vi "Main.vi"(11 "Module Admin":refnum<class "Delacor_lib_QMH_Module Admin.lvclass">) -> ()   [LabVIEW 2021, in "Control Panel.lvlib"]
doc: "This template is based off of the Queued Message Handler design pattern and the Queued Message Handler project template that ships with LabVIEW.\n\nThe main difference is that the queue is private to this module and communication between modules is performed via Broadcast and Request events.\n\nRequest events are wrapped in public API methods and are handled in the Event Handling Loop (EHL) of this VI. Any module can register for Broadcast events sent by this module. The EHL generates messages based on user interface actions.\n\nThe Message Handling Loop (MHL) processes messages generated by the EHL, or by other messages. The messages are string values, so new messages can be added easily to the Message Cases case structure in the MHL. Each message cluster can also provide an optional value for Message Data, which is a variant that can be converted to whatever message-specific data is required.\n_____\nBased on DQMH Project Template 7.0.1.1316."
uses:
  Control Panel.lvlib
  <vilib>/Delacor/Delacor QMH/Libraries/Message Queue_class/Delacor_lib_QMH_Message Queue.lvclass
  Module Data--cluster.ctl
  <vilib>/Delacor/Delacor QMH/Libraries/Message Queue_class/Delacor_lib_QMH_Enqueue Message (Single).vi
  Stop Argument--cluster.ctl
  <vilib>/Delacor/Delacor QMH/Libraries/Module Admin_class/Delacor_lib_QMH_Module Admin.lvclass
  PS/PS.lvlib
  DAQ/DAQ.lvlib
  SCOPE/SCOPE.lvlib
  Panel Load Argument--cluster.ctl
panel:
  in  "Options":i32(listbox)
  out "error out":errorcluster
  out "Status":string
  in  "Simulate MHL Error":bool
  in  "Simulate EHL Error":bool
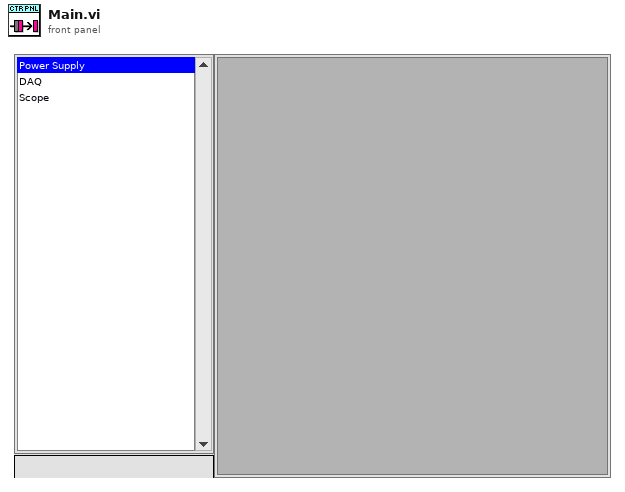
[diagram p1: front panel]
types:
  T1 = typedef "Control Panel.lvlib/Broadcast Events--cluster.ctl" = cluster{"Module Did Init":refnum<user-event>, "Status Updated":refnum<user-event>, "Error Reported":refnum<user-event>, "Module Did Stop":refnum<user-event>, "Update Module Execution Status":refnum<user-event>}
  T2 = typedef "PS.lvlib/Broadcast Events--cluster.ctl" = cluster{"Module Did Init":refnum<user-event>, "Status Updated":refnum<user-event>, "Error Reported":refnum<user-event>, "Module Did Stop":refnum<user-event>, "Update Module Execution Status":refnum<user-event>}
  T3 = typedef "DAQ.lvlib/Broadcast Events--cluster.ctl" = cluster{"Module Did Init":refnum<user-event>, "Status Updated":refnum<user-event>, "Error Reported":refnum<user-event>, "Module Did Stop":refnum<user-event>, "Update Module Execution Status":refnum<user-event>}
  T4 = typedef "SCOPE.lvlib/Broadcast Events--cluster.ctl" = cluster{"Module Did Init":refnum<user-event>, "Status Updated":refnum<user-event>, "Error Reported":refnum<user-event>, "Module Did Stop":refnum<user-event>, "Update Module Execution Status":refnum<user-event>}
  T5 = typedef "Control Panel.lvlib/Request Events--cluster.ctl" = cluster{"Stop Module":refnum<user-event>, "Show Panel":refnum<user-event>, "Hide Panel":refnum<user-event>, "Get Module Execution Status":refnum<user-event>, "Show Diagram":refnum<user-event>, "Private":cluster{"Panel Load":refnum<user-event>}}
  T6 = typedef "Control Panel.lvlib/Module Data--cluster.ctl" = cluster{"Status":string}
  T7 = enum32{"invalid lock state", "Not Locked", "Locked (No Password)", "Password-protected"}
  T8 = typedef "Control Panel.lvlib/Stop Argument--cluster.ctl" = cluster{"Origin":string, "Exit via Stop Module Req?":bool, "Wait for Module to stop?":bool}
  T9 = typedef "Control Panel.lvlib/Panel Load Argument--cluster.ctl" = cluster{"Panel Index":i32}
  T10 = enum32{"Invalid", "Standard", "Closed", "Hidden", "Minimized", "Maximized"}
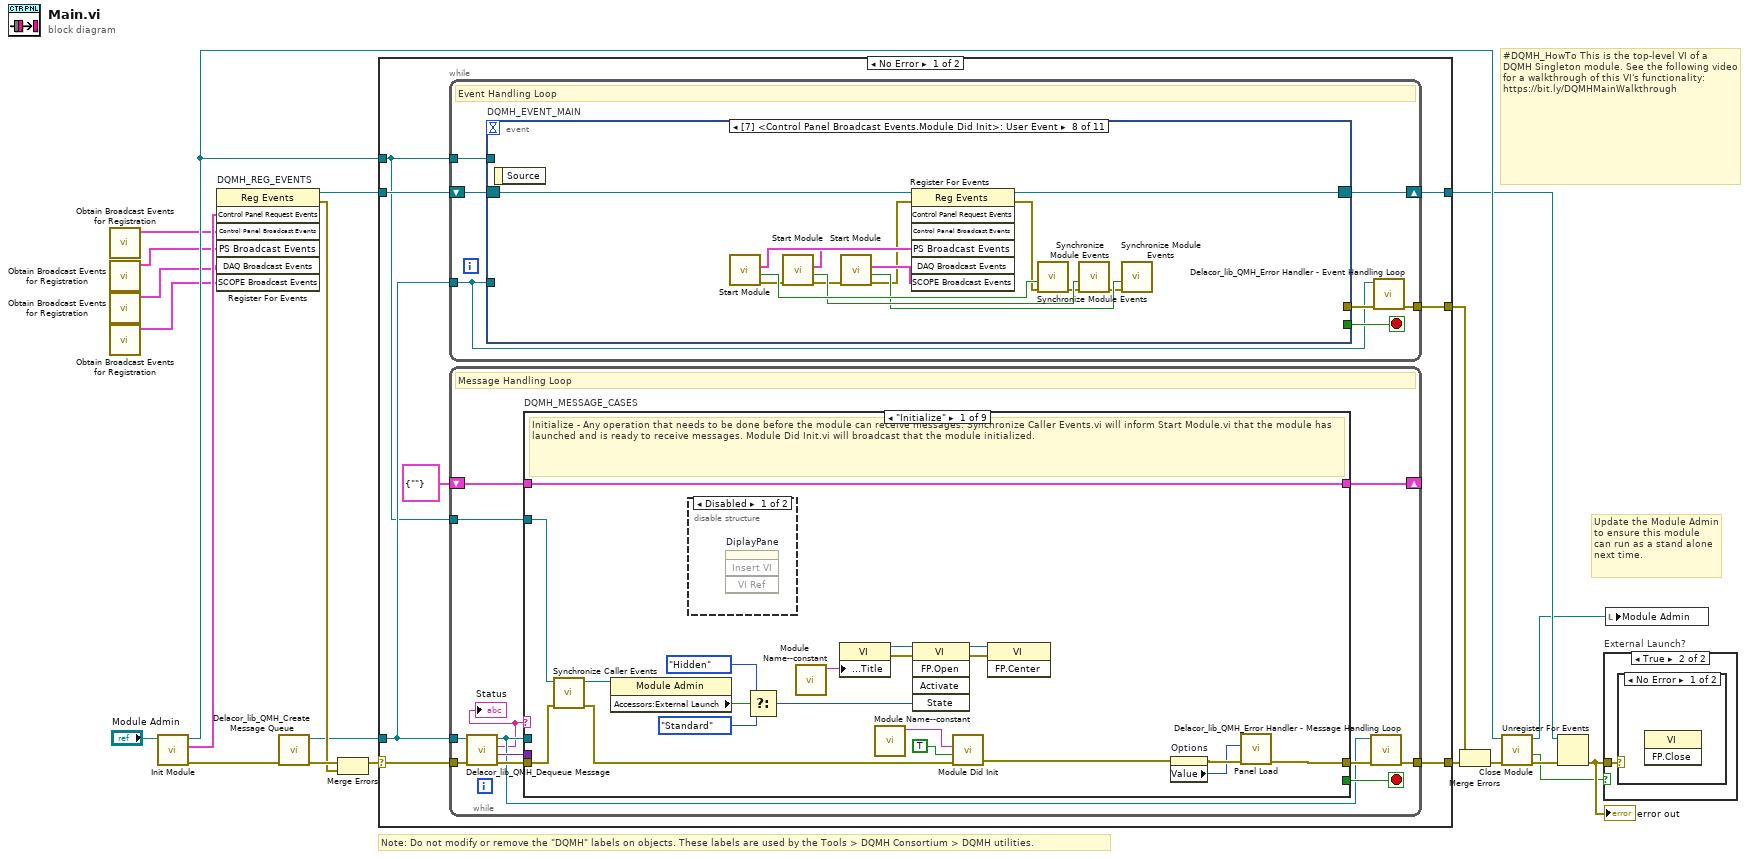
[diagram p0: block diagram]
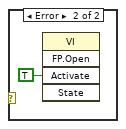
[diagram p3: hidden frame]
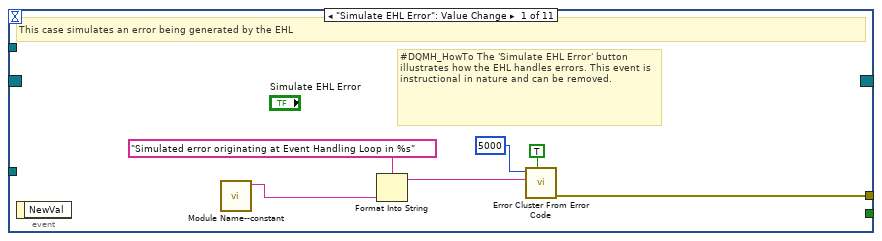
[diagram p4: hidden frame]
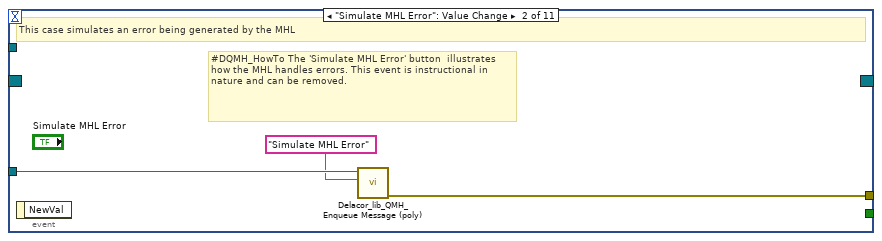
[diagram p5: hidden frame]
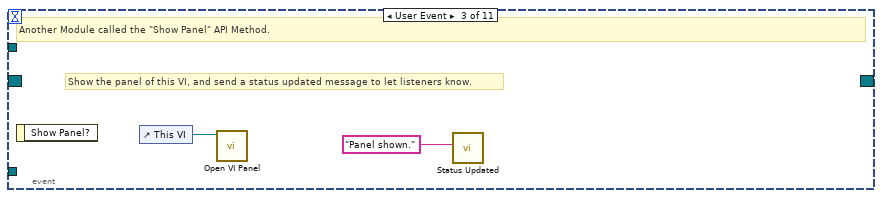
[diagram p6: hidden frame]
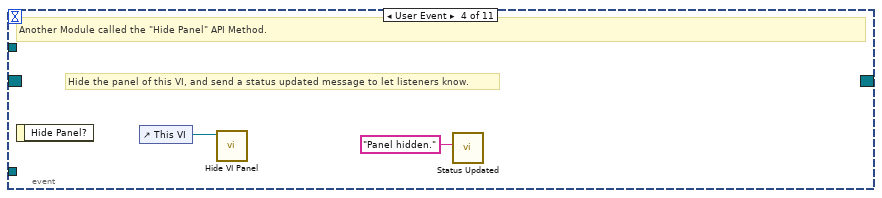
[diagram p7: hidden frame]
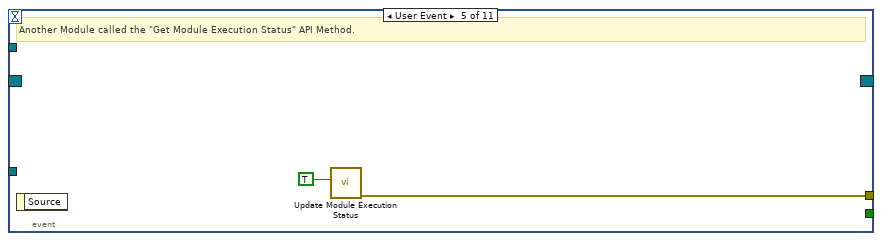
[diagram p8: hidden frame]
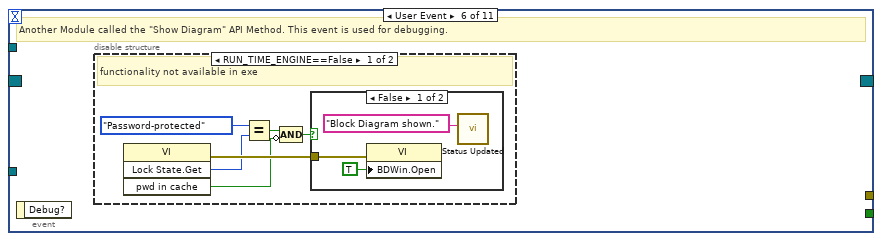
[diagram p9: hidden frame]
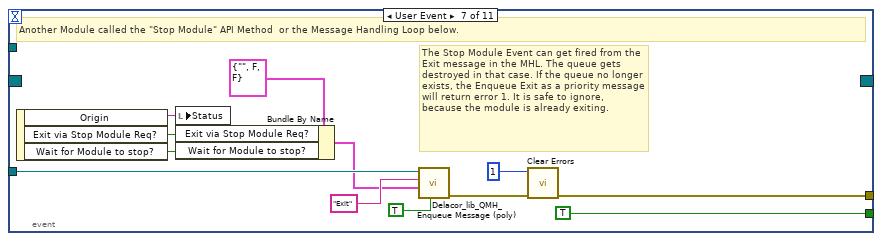
[diagram p12: hidden frame]
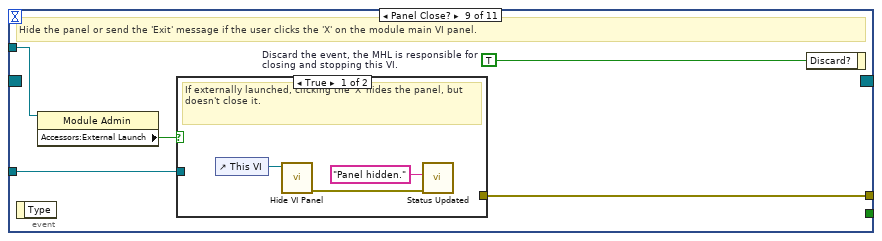
[diagram p13: hidden frame]
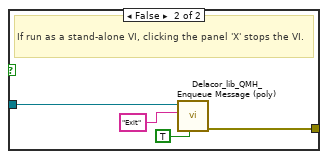
[diagram p14: hidden frame]
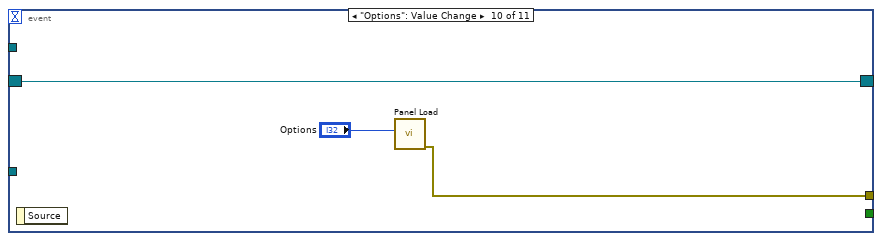
[diagram p15: hidden frame]
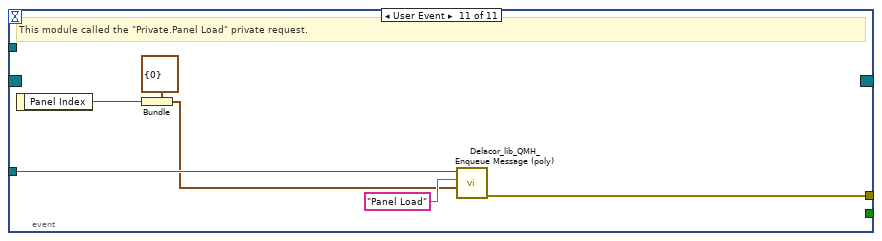
[diagram p16: hidden frame]
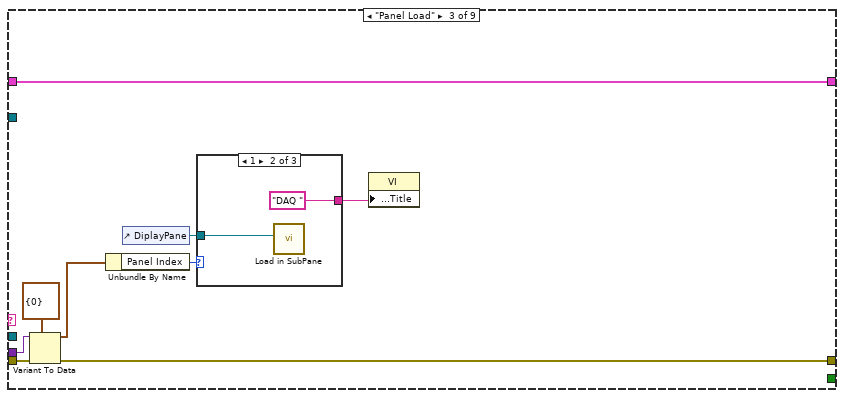
[diagram p19: hidden frame]
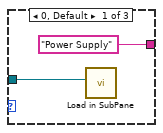
[diagram p20: hidden frame]
diagram:
  # "#DQMH_HowTo This is the top-level VI of a DQMH Singleton module. See the following video for a walkthrough of this VI's functionality: https://bit.ly/DQMHMainWalkthrough"
  # "Note: Do not modify or remove the \"DQMH\" labels on objects. These labels are used by the Tools > DQMH Consortium > DQMH utilities."
  # "Update the Module Admin to ensure this module can run as a stand alone next time."
  n1 = call "Obtain Broadcast Events for Registration.vi"() -> ("Control Panel Broadcast Events"=w4:T1)  [unwired: 9 in, 2 out]
  n2 = call "Obtain Broadcast Events for Registration.vi"() -> ("PS Broadcast Events"=w3:T2)  [unwired: 9 in, 2 out]
  n3 = call "Obtain Broadcast Events for Registration.vi"() -> ("DAQ Broadcast Events"=w2:T3)  [unwired: 9 in, 2 out]
  n4 = call "Obtain Broadcast Events for Registration.vi"() -> ("SCOPE Broadcast Events"=w1:T4)  [unwired: 9 in, 2 out]
  n5 = call "Init Module.vi"("Singleton Module Admin in"="Module Admin") -> ("error out"=w20:errorcluster, "Control Panel Request Events"=w9:T5, "Singleton Module Admin out"=w12:refnum<class "Delacor_lib_QMH_Module Admin.lvclass">)  [unwired: 8 in]
  n6 = register-events "DQMH_REG_EVENTS"(w9, w4, w3, w2, w1) -> (reference out=w10:refnum<event-registration>, error out=w13:errorcluster)  [unwired: 2 in]
  n7 = call <vilib>:"Delacor_lib_QMH_Create Message Queue.vi"("error in"=w20) -> ("error out"=w15:errorcluster, "Message Queue"=w8:refnum<class "Delacor_lib_QMH_Message Queue.lvclass">)  [unwired: 9 in]
  n8 = Merge Errors(w15, w13) -> (w14:errorcluster)
  n9 = case shown="No Error" w14 {
    selector: w14 -> [w27 w224]
    tunnel: [w29 w223] -> w21
    tunnel: [w26 w222] -> w11
    tunnel: w10 -> [w24 w222]
    tunnel: w8 -> [w23 w217]
    tunnel: [w28 _] -> w18
    tunnel: w12 -> [w22 w218]
    frame No Error {
      n10 = while {
        tunnel: w23 -> [w30]
        shift-right: [w33] -> w26
        shift-left: w24 -> [w34]
        tunnel: [w35] -> w28
        tunnel: w22 -> [w31]
        stop <- w32 stop-if-true
        # "Event Handling Loop"
        n11 = event "DQMH_EVENT_MAIN" shown="[7] <Control Panel Broadcast Events.Module Did Init>: User Event" {
          selector: w34 -> [_ _ _ _ _ _ _ w74 _ w101 _]
          dyn-events: [_ _ _ _ _ _ _ w73 _ w101 _] -> w33
          timeout: _ -> [_ _ _ _ _ _ _ _ _ _ _]
          tunnel: [_ _ _ _ _ _ TRUE ("Discard?") _ _ _ _] -> w32
          tunnel: w30 -> [_ w44 _ _ _ _ w68 _ w89 _ w107]
          tunnel: [w42 w45 _ _ w51 _ w71 _ w91 w99 w102] -> w36
          tunnel: w31 -> [_ _ _ _ _ _ _ _ w88 _ _]
          event "Simulate EHL Error": Value Change {
            # "#DQMH_HowTo The 'Simulate EHL Error' button  illustrates how the EHL handles errors. This event is instructional in nature and can be removed."
            # "This case simulates an error being generated by the EHL"
            n12 = event-data() -> ()  [unwired: 1 in, 1 out]
            n13 = call "Module Name--constant.vi"() -> ("Module Name"=w39:string)  [unwired: 11 in]
            n14 = Format Into String(format string="Simulated error originating at Event Handling Loop in %s", w39) -> (resulting string=w40:string)  [unwired: 2 in, 1 out]
            n15 = call <vilib>:"Error Cluster From Error Code.vi"("show call chain? (False)"=TRUE, "error message (\"\")"=w40, "error code (0)"=5000) -> ("error out"=w42:errorcluster)  [unwired: 6 in]
          }
          event "Simulate MHL Error": Value Change {
            # "#DQMH_HowTo The 'Simulate MHL Error' button  illustrates how the MHL handles errors. This event is instructional in nature and can be removed."
            # "This case simulates an error being generated by the MHL"
            n16 = event-data() -> ()  [unwired: 1 in, 1 out]
            n17 = call-poly <vilib>:"Delacor_lib_QMH_Enqueue Message (poly).vi"("Message"="Simulate MHL Error", "Message Queue in"=w44) -> ("error out"=w45:errorcluster)  [unwired: 8 in, 1 out]
          }
          event User Event {
            # "Show the panel of this VI, and send a status updated message to let listeners know."
            # "Another Module called the \"Show Panel\" API Method."
            n18 = event-data() -> ()  [unwired: 1 in, 1 out]
            n19 = control-ref of="This VI"() -> (w47:refnum<vi>)
            n20 = call "Open VI Panel.vi"("VI"=w47) -> ()  [unwired: 10 in, 1 out]
            n21 = call "Status Updated.vi"("Status"="Panel shown." ("format string")) -> ()  [unwired: 10 in, 1 out]
          }
          event User Event {
            # "Hide the panel of this VI, and send a status updated message to let listeners know."
            # "Another Module called the \"Hide Panel\" API Method."
            n22 = event-data() -> ()  [unwired: 1 in, 1 out]
            n23 = control-ref of="This VI"() -> (w49:refnum<vi>)
            n24 = call "Hide VI Panel.vi"("VI"=w49) -> ()  [unwired: 10 in, 1 out]
            n25 = call "Status Updated.vi"("Status"="Panel hidden." ("format string")) -> ()  [unwired: 10 in, 1 out]
          }
          event User Event {
            # "Another Module called the \"Get Module Execution Status\" API Method."
            n26 = event-data() -> ()  [unwired: 1 in, 1 out]
            n27 = call "Update Module Execution Status.vi"("Running?"=TRUE) -> ("error out"=w51:errorcluster)  [unwired: 10 in]
          }
          event User Event {
            # "Another Module called the \"Show Diagram\" API Method. This event is used for debugging."
            n28 = event-data() -> ()  [unwired: 1 in, 1 out]
            n29 = disable-structure shown="RUN_TIME_ENGINE==False" {
              frame condition #0 (active) {
                # "functionality not available in exe"
                n30 = invoke on="Invoke Node" class="VI" method="Lock State.Get"() -> (error out=w57:errorcluster, "Get Lock State"=w56:T7, "pwd in cache"=w53:bool)  [unwired: 4 in, 1 out]
                n31 = Equal?(x=T7."Password-protected", y=w56) -> (x = y?=w54:bool)
                n32 = Compound Arithmetic op=AND(w54, invert w53) -> (w52:bool)
                n33 = case shown="False" w52 {
                  tunnel: w57 -> [w60 _]
                  frame False {
                    n34 = property on="Property Node" class="VI"(error in=w60, "BDWin.Open"=TRUE ("Block Diagram Window:Open")) -> ()  [unwired: 1 in, 2 out]
                    n35 = call "Status Updated.vi"("Status"="Block Diagram shown." ("format string")) -> ()  [unwired: 10 in, 1 out]
                  }
                  frame True {
                    # "Password-protected VI, and the password is not in the cache. Do not show the diagram."
                  }
                }
              }
              frame condition #1 {
              }
            }
          }
          event User Event {
            # "The Stop Module Event can get fired from the Exit message in the MHL. The queue gets destroyed in that case. If the queue no longer exists, the Enqueue Exit as a priority message will return error 1. It is safe to ignore, because the module is already exiting."
            # "Another Module called the \"Stop Module\" API Method  or the Message Handling Loop below."
            n36 = event-data() -> ("Origin"=w67:string, "Exit via Stop Module Req?"=w63:bool, "Wait for Module to stop?"=w62:bool)  [unwired: 1 in]
            n37 = local write "Status"(w67) -> ()
            n38 = Bundle By Name(cluster=T8 {"Origin"="", "Exit via Stop Module Req?"=FALSE, "Wait for Module to stop?"=FALSE} ("Stop Argument"), "Exit via Stop Module Req?"=w63, "Wait for Module to stop?"=w62) -> (w61:T8)
            n39 = call-poly <vilib>:"Delacor_lib_QMH_Enqueue Message (poly).vi"("Priority Message? (F)"=TRUE, "Message Data"=w61, "Message"="Exit", "Message Queue in"=w68) -> ("error out"=w72:errorcluster)  [unwired: 6 in, 1 out]
            n40 = call <vilib>:"Clear Errors.vi"("error in (no error)"=w72, "specific error code to clear (0: all)"=1) -> ("error out"=w71:errorcluster)  [unwired: 4 in, 1 out]
          }
          event User Event {
            n41 = event-data() -> ()  [unwired: 1 in, 1 out]
            n42 = call "Start Module.vi"() -> ("error out"=w80:errorcluster, "Wait for Event Sync?"=w86:bool, "PS Broadcast Events"=w83:T2)  [unwired: 8 in, 1 out]
            n43 = call "Start Module.vi"("error in (no error)"=w80) -> ("error out"=w79:errorcluster, "Wait for Event Sync?"=w85:bool, "SCOPE Broadcast Events"=w82:T4)  [unwired: 7 in, 1 out]
            n44 = call "Start Module.vi"("error in (no error)"=w79) -> ("error out"=w78:errorcluster, "Wait for Event Sync?"=w84:bool, "DAQ Broadcast Events"=w81:T3)  [unwired: 7 in, 1 out]
            n45 = register-events(reference=w74, error in=w78, w83, w82, w81) -> (reference out=w73:refnum<event-registration>, error out=w77:errorcluster)  [unwired: 2 in]
            n46 = call "Synchronize Module Events.vi"("error in (no error)"=w77, "Wait for Event Sync?"=w86) -> ("error out"=w75:errorcluster)  [unwired: 9 in]
            n47 = call "Synchronize Module Events.vi"("error in (no error)"=w75, "Wait for Event Sync?"=w85) -> ("error out"=w76:errorcluster)  [unwired: 9 in]
            n48 = call "Synchronize Module Events.vi"("error in (no error)"=w76, "Wait for Event Sync?"=w84) -> ()  [unwired: 9 in, 1 out]
          }
          event Panel Close? {
            w90 = TRUE  # Discard the event, the MHL is responsible for closing and stopping this VI.
            # "Hide the panel or send the 'Exit' message if the user clicks the 'X' on the module main VI panel."
            n49 = event-data() -> ()  [unwired: 1 in, 1 out]
            n50 = property on="Property Node" class="Module Admin"(reference=w88) -> ("Accessors:External Launch"=w87:bool)  [unwired: 1 in, 2 out]
            n51 = case shown="True" w87 {
              tunnel: w89 -> [_ w97]
              tunnel: [_ w98] -> w91
              frame True {
                # "If externally launched, clicking the 'X' hides the panel, but doesn't close it."
                n52 = control-ref of="This VI"() -> (w94:refnum<vi>)
                n53 = call "Hide VI Panel.vi"("VI"=w94) -> ("error out"=w92:errorcluster)  [unwired: 10 in]
                n54 = call "Status Updated.vi"("error in"=w92, "Status"="Panel hidden." ("format string")) -> ()  [unwired: 9 in, 1 out]
              }
              frame False {
                # "If run as a stand-alone VI, clicking the panel 'X' stops the VI."
                n55 = call-poly <vilib>:"Delacor_lib_QMH_Enqueue Message (poly).vi"("Priority Message? (F)"=TRUE, "Message"="Exit", "Message Queue in"=w97) -> ("error out"=w98:errorcluster)  [unwired: 7 in, 1 out]
              }
            }
            n56 = event-data ("Event Filter Node")("Discard?"=w90) -> ()  [unwired: 1 in, 1 out]
          }
          event "Options": Value Change {
            n57 = event-data() -> ()  [unwired: 1 in, 1 out]
            n58 = call "Panel Load.vi"("Panel Index"="Options") -> ("error out"=w99:errorcluster)  [unwired: 10 in]
          }
          event User Event {
            # "This module called the \"Private.Panel Load\" private request."
            n59 = event-data() -> ("Panel Index"=w103:i32)  [unwired: 1 in]
            n60 = Bundle(cluster=T9 {"Panel Index"=0} ("Panel Load Argument"), "Panel Index"=w103) -> (w104:T9)
            n61 = call-poly <vilib>:"Delacor_lib_QMH_Enqueue Message (poly).vi"("Message Data"=w104, "Message"="Panel Load", "Message Queue in"=w107) -> ("error out"=w102:errorcluster)  [unwired: 7 in, 1 out]
          }
        }
        n62 = call-dynamic "Delacor_lib_QMH_Error Handler - Event Handling Loop.vi"("error in"=w36, "Message Queue in"=w30) -> ("dup error in"=w35:errorcluster)  [unwired: 8 in, 1 out]
      }
      n63 = while {
        tunnel: w23 -> [w109]
        shift-right: [w116] -> _
        shift-left: T6 {"Status"=""} ("Data Cluster") -> [w117]
        tunnel: w27 -> [w119]
        tunnel: [w112] -> w29
        tunnel: w22 -> [w113]
        stop <- w115 stop-if-true
        # "Message Handling Loop"
        n64 = call-dynamic "Delacor_lib_QMH_Dequeue Message.vi"("error in"=w119, "Message Queue in"=w109) -> ("error out"=w118:errorcluster, "Message Data"=w114:variant, "Message"=w108:string, "Message Queue out"=w110:refnum<class "Delacor_lib_QMH_Message Queue.lvclass">)  [unwired: 6 in]
        "Status" <- w108
        n65 = case "DQMH_MESSAGE_CASES" shown="\"Initialize\"" w108 {
          selector: w108 -> [_ _ _ _ _ _ _ _ w212]
          tunnel: w110 -> [_ _ _ _ _ _ w174 w200 _]
          tunnel: w118 -> [w137 w141 w150 w159 w161 w170 w181 w206 w215]
          tunnel: [w123 w141 w148 w158 w161 w169 w177 w201 w216] -> w111
          tunnel: w117 -> [w124 w140 w149 w157 w160 w167 w176 w199 w213]
          tunnel: [w124 w140 w149 w157 w160 w167 w176 w199 w213] -> w116
          tunnel: [_ _ _ _ _ _ _ w198 _] -> w115
          tunnel: w114 -> [_ _ w147 _ _ _ w175 w197 _]
          tunnel: w113 -> [w128 _ _ _ _ _ w173 w192 _]
          frame "Initialize" {
            # "Initialize - Any operation that needs to be done before the module can receive messages. Synchronize Caller Events.vi will inform Start Module.vi that the module has launched and is ready to receive messages. Module Did Init.vi will broadcast that the module initialized."
            n66 = call "Synchronize Caller Events.vi"("error in"=w137, "Singleton Module Admin in"=w128) -> ("error out"=w136:errorcluster, "Singleton Module Admin out"=w125:refnum<class "Delacor_lib_QMH_Module Admin.lvclass">)  [unwired: 8 in]
            n67 = property on="Property Node" class="Module Admin"(reference=w125) -> ("Accessors:External Launch"=w132:bool)  [unwired: 1 in, 2 out]
            n68 = disable-structure shown="Disabled" {
              frame Disabled {
                n69 = invoke on="DiplayPane" class="SubPnl" method="Insert VI"() -> ()  [unwired: 4 in, 4 out]
              }
              frame Enabled {
              }
            }
            n70 = Select(t=T10."Hidden" ("State"), s=w132, f=T10."Standard" ("State")) -> (s? t:f=w129:T10)
            n71 = call "Module Name--constant.vi"() -> ("Module Name"=w135:string)  [unwired: 11 in]
            n72 = property on="Property Node" class="VI"("Front Panel.Title"=w135) -> (reference out=w134:refnum<vi>, error out=w139:errorcluster)  [unwired: 2 in]
            n73 = call "Module Name--constant.vi"() -> ("Module Name"=w126:string)  [unwired: 11 in]
            n74 = invoke on="Invoke Node" class="VI" method="FP.Open"(reference=w134, error in=w139, "State"=w129) -> (reference out=w133:refnum<vi>, error out=w138:errorcluster)  [unwired: 2 in, 3 out]
            n75 = call "Module Did Init.vi"("error in"=w136, "Initialized?"=TRUE, "Origin"=w126) -> ("error out"=w122:errorcluster)  [unwired: 8 in]
            n76 = invoke on="Invoke Node" class="VI" method="FP.Center"(reference=w133, error in=w138) -> ()  [unwired: 1 in, 3 out]
            n77 = property on="Options" class="LstBox (strict)"(error in=w122) -> (error out=w121:errorcluster, "Value"=w120:i32)  [unwired: 1 in, 1 out]
            n78 = call "Panel Load.vi"("error in"=w121, "Panel Index"=w120) -> ("error out"=w123:errorcluster)  [unwired: 9 in]
          }
          frame "---Module Specific---" {
            # "Separator -- The following cases handle messages specific to this Module."
          }
          frame "Panel Load" {
            n79 = Variant To Data(error in=w150, type=T9 {"Panel Index"=0} ("Panel Load Argument"), Variant=w147) -> (data=w145:T9, error out=w148:errorcluster)
            n80 = Unbundle By Name(w145) -> ("Panel Index"=w144:i32)
            n81 = control-ref of="DiplayPane"() -> (w143:refnum<vi>)
            n82 = case shown="1" w144 {
              tunnel: w143 -> [w152 w154 w156]
              tunnel: ["Power Supply" "DAQ " "SCOPE"] -> w142
              frame 0, Default {
                n83 = call "Load in SubPane.vi"("Subpanel Ref"=w152) -> ()  [unwired: 10 in, 1 out]
              }
              frame 1 {
                n84 = call "Load in SubPane.vi"("Subpanel Ref"=w154) -> ()  [unwired: 10 in, 1 out]
              }
              frame 2 {
                n85 = call "Load in SubPane.vi"("Subpanel Ref"=w156) -> ()  [unwired: 10 in, 1 out]
              }
            }
            n86 = property on="Property Node" class="VI"("Front Panel.Title"=w142) -> ()  [unwired: 2 in, 2 out]
          }
          frame "---Copy This Frame---" {
            # "Duplicate this frame when creating new messages.  Change this comment in the duplicated frame to describe this message."
            n87 = Merge Errors(w159) -> (w158:errorcluster)
          }
          frame "---Exit and Error Handling---" {
            # "Separator - The following cases handle errors and exit messages."
          }
          frame "Simulate MHL Error" {
            # "#DQMH_HowTo The 'Simulate MHL Error' button  illustrates how the MHL handles errors. This event is instructional in nature and can be removed."
            # "Simulate an error occurring at the MHL"
            n88 = call "Module Name--constant.vi"() -> ("Module Name"=w163:string)  [unwired: 11 in]
            n89 = Format Into String(format string="Simulated error originating at Message Handling Loop in %s", w163) -> (resulting string=w164:string)  [unwired: 2 in, 1 out]
            n90 = call <vilib>:"Error Cluster From Error Code.vi"("show call chain? (False)"=TRUE, "error message (\"\")"=w164, "error code (0)"=5001) -> ("error out"=w168:errorcluster)  [unwired: 6 in]
            n91 = Merge Errors(w170, w168) -> (w169:errorcluster)
          }
          frame "Error" {
            # "#CodeRecommended - If the module is running in standalone mode (External Launch = FALSE), this code will pop up an error dialog and call the 'Exit' message if an error occurs. Add more fine-grained error management here."
            # "Error - Check the error message data and respond accordingly. This message is sent by the \"Error Handler\" VIs at the end of each loop in this application."
            n92 = property on="Property Node" class="Module Admin"(reference=w173) -> ("Accessors:External Launch"=w172:bool)  [unwired: 1 in, 2 out]
            n93 = Variant To Data(error in=w181, type=errorcluster {"status"=FALSE, "code"=0, "source"=""} ("error constant"), Variant=w175) -> (data=w171:errorcluster, error out=w179:errorcluster)
            n94 = local write "error out"(w171) -> ()
            n95 = call "Error Reported.vi"("Error"=w171) -> ()  [unwired: 10 in, 1 out]
            n96 = case shown="False" w172 {
              tunnel: [w186 _] -> w178
              tunnel: w174 -> [w184 _]
              tunnel: w171 -> [w185 _]
              frame False {
                n97 = disable-structure shown="Default" {
                  disable-tunnel: w185 -> [w187 _]
                  frame condition #0 (active) {
                    # "If the module is running standalone, then pop up an error dialog and call the \"Exit\" message."
                    n98 = call <vilib>:"Simple Error Handler.vi"("error in (no error)"=w187) -> ()  [unwired: 4 in, 5 out]
                  }
                  frame condition #1 {
                    # "To prevent the Simple Error Handler VI from being loaded (e.g. when deploying to a Real-Time target), add the Conditional Disable Symbol \"DQMH_Disable_SEH\" to your project and set it to TRUE."
                  }
                }
                n99 = call-poly <vilib>:"Delacor_lib_QMH_Enqueue Message (poly).vi"("Priority Message? (F)"=TRUE, "Message"="Exit", "Message Queue in"=w184) -> ("error out"=w186:errorcluster)  [unwired: 7 in, 1 out]
              }
              frame True {
                # "If the module was launched externally, calling the Error Reported broadcast VI is the only action performed by the \"Error\" message. The module's caller can then process the error appropriately."
              }
            }
            n100 = Merge Errors(w179, w178) -> (w177:errorcluster)
          }
          frame "Exit" {
            w196 = 91  # 91: not all Exit messages will have an argument
            w198 = TRUE  # Stop the VI
            # "Release the message queue reference"
            # "#CodeNeeded - Add any required cleanup code here."
            # "Exit - Exit the application."
            n101 = Variant To Data(error in=w206, type=T8 {"Origin"="", "Exit via Stop Module Req?"=FALSE, "Wait for Module to stop?"=FALSE} ("Stop Argument"), Variant=w197) -> (data=w194:T8, error out=w203:errorcluster)
            n102 = call "Stop Module.vi"() -> ("error out"=w191:errorcluster)  [unwired: 11 in]
            n103 = call <vilib>:"Clear Errors.vi"("error in (no error)"=w203, "specific error code to clear (0: all)"=w196) -> ("error out"=w205:errorcluster)  [unwired: 4 in, 1 out]
            n104 = call "Stop Module.vi"() -> ("error out"=w190:errorcluster)  [unwired: 11 in]
            n105 = call "Stop Module.vi"() -> ("error out"=w189:errorcluster)  [unwired: 11 in]
            n106 = control-ref of="This VI"() -> (w193:refnum<vi>)
            n107 = Merge Errors(w189, w190, w191) -> (w188:errorcluster)
            n108 = call-dynamic "Delacor_lib_QMH_Release Message Queue.vi"("error in"=w205, "Message Queue"=w200) -> ("error out"=w204:errorcluster)  [unwired: 9 in]
            n109 = call "Handle Exit.vi"("error in"=w188, "Stop Argument"=w194, "Admin in"=w192, "VI reference"=w193) -> ("error out"=w202:errorcluster)  [unwired: 6 in, 1 out]
            n110 = Merge Errors(w204, w202) -> (w201:errorcluster)
            n111 = call "Error Reported.vi"("Error"=w201) -> ()  [unwired: 10 in, 1 out]
          }
          frame Default {
            # "'Default' case only runs if there is a message that isn't defined in any of the other cases.  Output a programming error."
            n112 = call "Module Name--constant.vi"() -> ("Module Name"=w211:string)  [unwired: 11 in]
            n113 = Format Into String(format string="The invalid message string \"%s\" was received in the Message Handling Loop for module \"%s\".", w212, w211) -> (resulting string=w207:string)  [unwired: 2 in, 1 out]
            n114 = call <vilib>:"Error Cluster From Error Code.vi"("show call chain? (False)"=TRUE, "error message (\"\")"=w207, "error code (0)"=1) -> ("error out"=w214:errorcluster)  [unwired: 6 in]
            n115 = Merge Errors(w215, w214) -> (w216:errorcluster)
          }
        }
        n116 = call-dynamic "Delacor_lib_QMH_Error Handler - Message Handling Loop.vi"("error in"=w111, "Message Queue in"=w110) -> ("dup error in"=w112:errorcluster)  [unwired: 8 in, 1 out]
      }
    }
    frame Error {
      # "Synchronize Caller Events.vi will inform Start Module.vi that the module has launched and will let the code calling Start Module.vi register for broadcasts and would permit the caller receive the broadcast that an error occurred at launch time."
      n117 = call-dynamic "Delacor_lib_QMH_Release Message Queue.vi"("error in"=w224, "Message Queue"=w217) -> ("error out"=w223:errorcluster)  [unwired: 9 in]
      n118 = call "Synchronize Caller Events.vi"("Singleton Module Admin in"=w218) -> ("error out"=w225:errorcluster)  [unwired: 9 in, 1 out]
      n119 = call "Module Name--constant.vi"() -> ("Module Name"=w221:string)  [unwired: 11 in]
      n120 = Format Into String(format string="An error occurred during initialization. %s is no longer running.", w221) -> (resulting string=w219:string)  [unwired: 2 in, 1 out]
      n121 = Merge Errors(w223, w225) -> (w226:errorcluster)
      n122 = call "Error Reported.vi"("Additional Information"=w219, "Error"=w226) -> ()  [unwired: 9 in, 1 out]
    }
  }
  n123 = Merge Errors(w18, w21) -> (w17:errorcluster)
  n124 = call "Close Module.vi"("error in"=w17, "Module Admin in"=w12) -> ("error out"=w19:errorcluster, "External Launch"=w5:bool, "Module Admin out"=w6:refnum<class "Delacor_lib_QMH_Module Admin.lvclass">)  [unwired: 7 in]
  n125 = Unregister For Events(event registration refnum=w11, error in=w19) -> (error out=w16:errorcluster)
  "error out" <- w16
  n126 = case "External Launch?" shown="True" w5 {
    tunnel: w16 -> [_ w227]
    frame False {
    }
    frame True {
      n127 = case shown="No Error" w227 {
        frame No Error {
          n128 = invoke on="Invoke Node" class="VI" method="FP.Close"() -> ()  [unwired: 3 in, 3 out]
        }
        frame Error {
          n129 = invoke on="Invoke Node" class="VI" method="FP.Open"("Activate"=TRUE ("Activate?")) -> ()  [unwired: 4 in, 5 out]
        }
      }
    }
  }
  n130 = local write "Module Admin"(w6) -> ()
